vi "Invoke Container.vi"(8 "error in (no error)":errorcluster, 10 "Container":refnum<vi>, 11 "Generic Item in":refnum<class "Generic Item.lvclass">) -> (0 "error out":errorcluster, 3 "Generic Item out":refnum<class "Generic Item.lvclass">)   [LabVIEW 2015, in "Item Actor.lvlib" / "Generic Item.lvclass"]
uses:
  Generic Item.lvclass
  Generic Item.lvclass/Generic Item.ctl
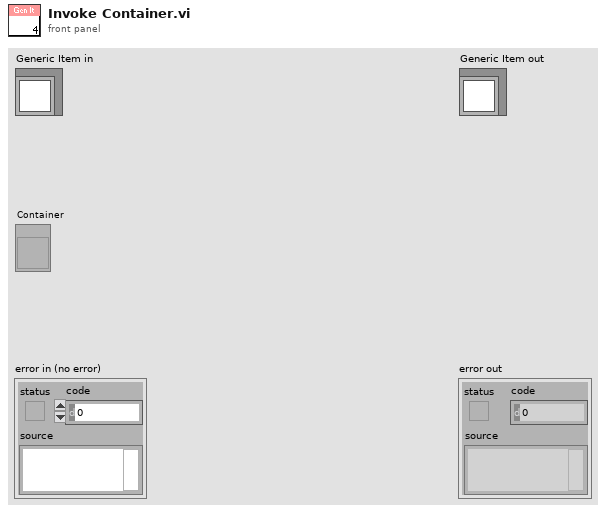
[diagram p1: front panel]
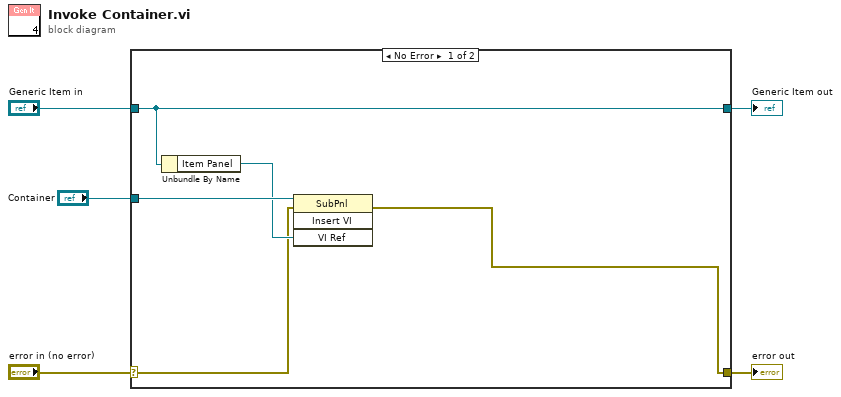
[diagram p0: block diagram]
diagram:
  n1 = case shown="No Error" "error in (no error)" {
    selector: "error in (no error)" -> [w6 w12]
    tunnel: [w7 w12] -> w4
    tunnel: [w10 w11] -> w2
    tunnel: "Generic Item in" -> [w10 w11]
    tunnel: "Container" -> [w9 _]
    frame No Error {
      n2 = Unbundle By Name(w10) -> ("Item Panel"=w8:refnum<vi>)
      n3 = invoke class="SubPnl" method="Insert VI"(reference=w9, error in=w6, "VI Ref"=w8) -> (error out=w7:errorcluster)  [unwired: 1 in, 3 out]
    }
    frame Error {
    }
  }
  "error out" <- w4
  "Generic Item out" <- w2
